vi "Get Topology.vi"(0 "SLSC Switch in":refnum<class "SLSC Switch.lvclass">, 5 "Topology Name In":string, 11 "error in (no error)":errorcluster) -> (4 "SLSC Switch out":refnum<class "SLSC Switch.lvclass">, 6 "Topology Name Out":string, 8 "Topology File Path out":path, 10 "Active Index":i32, 15 "error out":errorcluster)   [LabVIEW 2015, in "SLSC Switch.lvclass"]
uses:
  SLSC Switch.lvclass
  SLSC Switch.lvclass/SLSC Switch.ctl
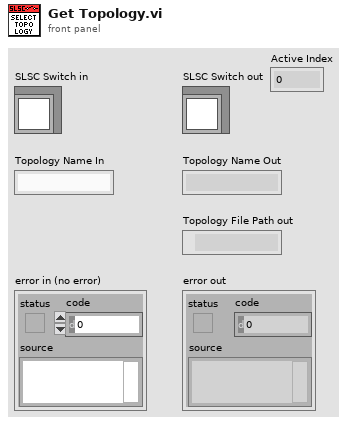
[diagram p1: front panel]
types:
  T1 = typedef "SLSC Switch.lvclass/Topology.ctl" = cluster{"Topology Name":string, "Topology File Path":path, "Channels":string[]}
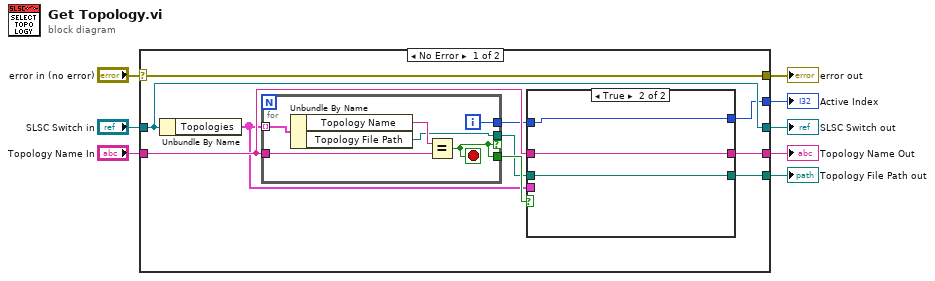
[diagram p0: block diagram]
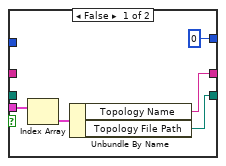
[diagram p2: hidden frame]
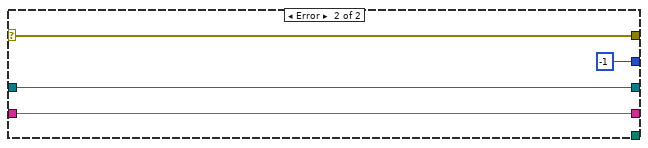
[diagram p3: hidden frame]
diagram:
  n1 = case shown="No Error" "error in (no error)" {
    selector: "error in (no error)" -> [w12 w36]
    tunnel: [w12 w36] -> w7
    tunnel: [w18 w35] -> w5
    tunnel: "SLSC Switch in" -> [w18 w35]
    tunnel: "Topology Name In" -> [w13 w33]
    tunnel: [w16 _] -> w3
    tunnel: [w14 w33] -> w2
    tunnel: [w9 -1] -> w1
    frame No Error {
      n2 = Unbundle By Name(w18) -> ("Topologies"=w11:T1[])
      n3 = for {
        tunnel: w11 -> [w32] mode=indexing
        tunnel: w13 -> [w30]
        tunnel: [w29] -> w15 if=w28
        tunnel: [w28] -> w17
        tunnel: [w27] -> w10
        i -> [w27]
        stop <- w28 stop-if-true
        n4 = Unbundle By Name(w32) -> ("Topology Name"=w31:string, "Topology File Path"=w29:path)
        n5 = Equal?(x=w31, y=w30) -> (x = y?=w28:bool)
      }
      n6 = case shown="True" w17 {
        tunnel: [w21 w26] -> w16
        tunnel: w15 -> [_ w26]
        tunnel: [w22 w25] -> w14
        tunnel: w13 -> [_ w25]
        tunnel: w11 -> [w23 _]
        tunnel: w10 -> [_ w24]
        tunnel: [0 w24] -> w9
        frame False {
          n7 = Index Array(array=w23) -> (element=w20:T1)  [unwired: 1 in]
          n8 = Unbundle By Name(w20) -> ("Topology Name"=w22:string, "Topology File Path"=w21:path)
        }
        frame True {
        }
      }
    }
    frame Error {
    }
  }
  "error out" <- w7
  "SLSC Switch out" <- w5
  "Topology File Path out" <- w3
  "Topology Name Out" <- w2
  "Active Index" <- w1
